vi "Get DDGIOC Pulses.vi"(11 "pulses":i32) -> (2 "function return":u32, 3 "pulses out":i32)   [LabVIEW 2018, in "AndorSDK.lvlib"]
doc: "EXPNETTYPE unsigned int WINAPI GetDDGIOCPulses(int * pulses);"
uses:
  AndorSDK.lvlib
  ATMCD32D.dll
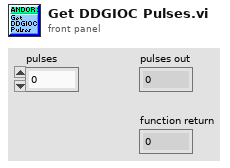
[diagram p1: front panel]
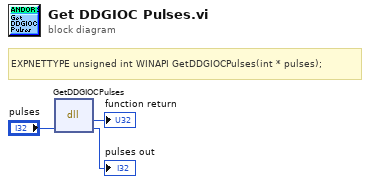
[diagram p0: block diagram]
diagram:
  # "EXPNETTYPE unsigned int WINAPI GetDDGIOCPulses(int * pulses);"
  n1 = dll-call lib="PTH2babs E\nPersönliches02 - Arbeit03-HiwijobsLabviewCodelibANDOR\tAndor SDK\nATMCD32D.*" fn="GetDDGIOCPulses"("pulses"="pulses") -> (→"function return":u32, "pulses"=→"pulses out":i32)  [unwired: 3 in, 2 out]
